vi "GetTextDimension.vi"(8 "error in (no error)":errorcluster, 10 "Name":string, 11 "LcPictureBox in":refnum<class "LcPictureBox.lvclass">) -> (0 "error out":errorcluster, 1 "TextSize(Pts)":dbl, 2 "Height":sgl, 3 "Width":sgl)   [LabVIEW 2020, in "LcPictureBox.lvclass"]
uses:
  LcPictureBox.lvclass
  SmoothingMode.ctl
  Font.ctl
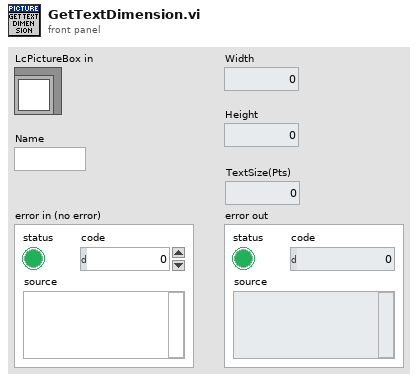
[diagram p1: front panel]
types:
  T1 = typedef "LcPictureBox.lvclass/Font.ctl" = cluster{"FontName":string, "Size(Pts)":dbl, "Style":enum16{"Regular", "Bold", "Italic", "Underline", "Strikeout"}}
  T2 = typedef "LcPictureBox.lvclass/SmoothingMode.ctl" = enum16{"None", "HighSpeed", "HighQuality", "AntiAlias"}
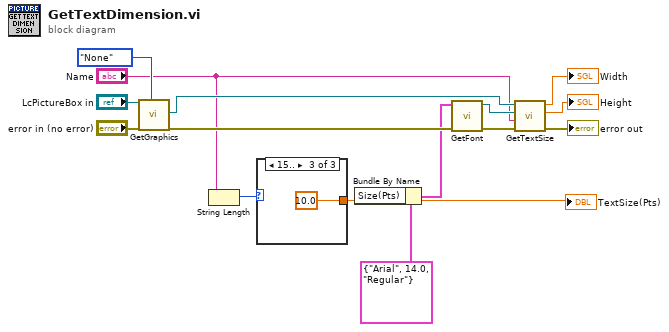
[diagram p0: block diagram]
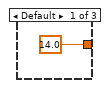
[diagram p2: hidden frame]
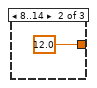
[diagram p3: hidden frame]
diagram:
  n1 = call "GetGraphics.vi"("LcPictureBox in"="LcPictureBox in", "error in (no error)"="error in (no error)", "SmoothingMode"=SmoothingMode."None") -> ("Graphics"=w10:refnum<k24>, "error out"=w7:errorcluster)  [unwired: 12 in, 3 out]
  n2 = String Length(string="Name") -> (length=w2:i32)
  n3 = case shown="15.." w2 {
    tunnel: [14.0 ("Size(Pts)") 12.0 ("Size(Pts)") 10.0 ("Size(Pts)")] -> w1
    frame Default {
    }
    frame 8..14 {
    }
    frame 15.. {
    }
  }
  "TextSize(Pts)" <- w1
  n4 = Bundle By Name(cluster=T1 {"FontName"="Arial", "Size(Pts)"=14.0, "Style"=enum."Regular"} ("Font(Arial,14pts,Regular)"), "Size(Pts)"=w1) -> (w3:T1)
  n5 = call "GetFont.vi"("error in (no error)"=w7, "Font(Arial,14pts,Regular)"=w3) -> ("error out"=w8:errorcluster, "Font"=w9:refnum<k24>)  [unwired: 8 in]
  n6 = call "GetTextSize.vi"("Error In"=w8, "Text"="Name", "Font"=w9, "Graphics"=w10) -> ("Error Out"=→"error out":errorcluster, "Height"=→"Height":sgl, "Width"=→"Width":sgl)  [unwired: 5 in]
